vi "TEST Registry With Units.vi"() -> ()   [LabVIEW 2013, in "Carya Config.lvclass"]
doc: "Copyright 2018, Carya Automatisering, Wiebe Walstra."
uses:
  Carya Config.lvclass
  CConfig Variant Accessor/CConfig Variant Accessor.lvclass
  <vilib>/Utility/VariantDataType/VariantType.lvlib
panel:
  out "data 2":csg
  out "variant 2":variant
  out "variant":variant
  out "Formatted Strings 2":string[](array[string])
  out "x 2":dbl
  out "x":dbl
  out "J Bevel_cap height (m)":dbl[unit]
  out "J Bevel_cap height (m)":dbl=1.0
  in  "J Bevel_cap height (m)":dbl[unit]=0.001
  out "String 2":string
  out "Formatted Strings":string[](array[string])
  out "Numeric":cxt
  out "data":T1
  out "error out":errorcluster
  out "String":string
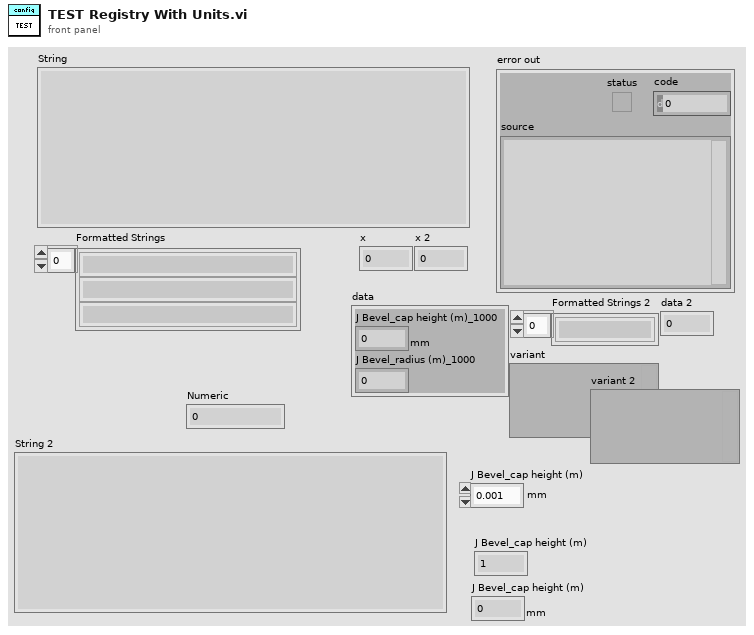
[diagram p1: front panel]
types:
  T1 = cluster{"J Bevel_cap height (m)_1000":dbl[unit], "J Bevel_radius (m)_1000":dbl}
  T2 = cluster{"J Bevel_cap height (m)_1000":dbl[unit], "J Bevel_cap height (m)_1000 2":dbl[unit], "J Bevel_cap height (m)_1000 3":dbl[unit]}
  T3 = cluster{"J Bevel_cap height (m)_1000":dbl, "J Bevel_radius (m)_1000":dbl}
  T4 = typedef "VariantType.lvlib/UnitInfo.ctl" = cluster{"UnitType":T5, "Exponent":i16}
  T5 = typedef "VariantType.lvlib/UnitType.ctl" = enum16{"Radians", "Steradians", "Seconds", "Meters", "Kilograms", "Amperes", "Kelvins", "Moles", "Candelas", "InvalidUnit"}
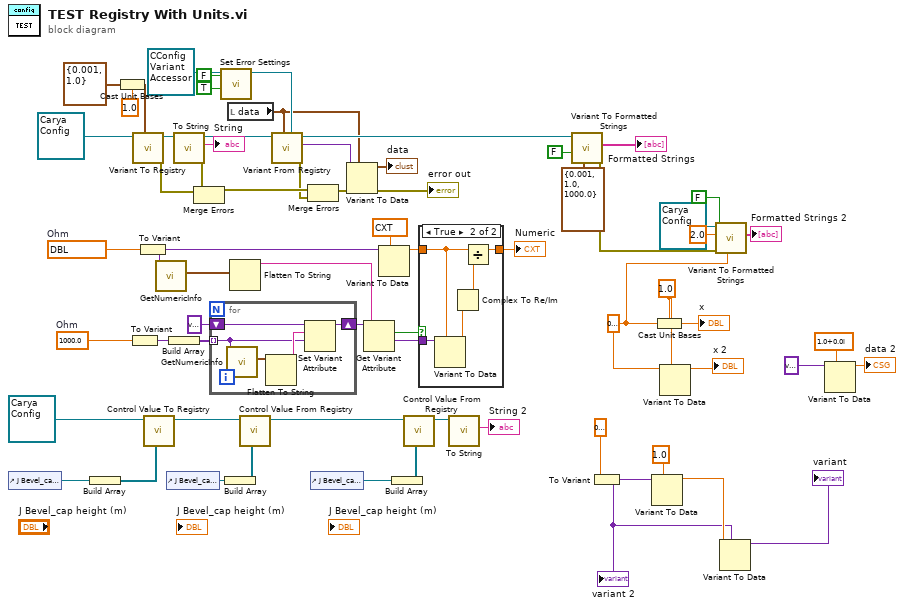
[diagram p0: block diagram]
diagram:
  w17 = 1.0 ("unit (none)")
  w15 = dbl[unit] 0.001 ("J Bevel_cap height (m)")
  w37 = dbl[unit] 1000.0  # Ohm
  w46 = cxt[unit] 100.0+200.0i  # Ohm
  n1 = control-ref of="J Bevel_cap height (m)"() -> (w29:refnum<vi>)
  n2 = Build Array(w29) -> (w28:refnum<vi>[])
  n3 = Cast Unit Bases(0:T1 {"J Bevel_cap height (m)_1000"=0.001, "J Bevel_radius (m)_1000"=1.0} ("J weld bevel"), 1:1.0) -> (2:w21:T3)
  n4 = To Variant(anything=w37) -> (Variant=w45:variant)
  n5 = call "Variant To Registry.vi"("Variant"=w21, "Carya Config in"=refnum<class "Carya Config.lvclass"> refnum) -> ("error out"=w62:errorcluster, "Carya Config out"=w66:refnum<class "Carya Config.lvclass">)  [unwired: 6 in, 2 out]
  n6 = To Variant(anything=w46) -> (Variant=w44:variant)
  n7 = call "Control Value To Registry.vi"("Controls"=w28, "Registry Object in"=refnum<class "Carya Config.lvclass"> refnum ("Carya Config in")) -> ("Registry Object out"=w30:refnum<class "Carya Config.lvclass">)  [unwired: 5 in, 4 out]
  n8 = call <vilib>:"GetNumericInfo.vi"("Variant"=w44) -> ("Units"=w41:T4[])  [unwired: 7 in, 3 out]
  n9 = control-ref of="J Bevel_cap height (m)"() -> (w27:refnum<vi>)
  n10 = Build Array(w45) -> (w47:variant[])
  n11 = call-dynamic "To String.vi"("Carya Config in"=w66) -> ("error out"=w63:errorcluster, "String"=→"String":string, "Carya Config out"=w64:refnum<class "Carya Config.lvclass">)  [unwired: 8 in]
  n12 = Merge Errors(w62, w63) -> (w61:errorcluster)
  n13 = for {
    tunnel: w47 -> [w69] mode=indexing
    shift-right: [w67] -> w42
    shift-left: variant -> [w68]
    n14 = call <vilib>:"GetNumericInfo.vi"("Variant"=w69) -> ("Units"=w71:T4[])  [unwired: 7 in, 3 out]
    n15 = Flatten To String(anything=w71) -> (data string=w70:string)  [unwired: 3 in, 2 out]
    n16 = Set Variant Attribute(Variant=w68, name=w70, value=w69) -> (Variant out=w67:variant)  [unwired: 1 in, 2 out]
  }
  n17 = call "Set Error Settings.vi"("Key not found error [F]"=TRUE ("Key not found error [T]"), "Wrong label error [F]"=FALSE, "CConfig Variant Accessor in"=refnum<class "CConfig Variant Accessor.lvclass"> refnum) -> ("CConfig Variant Accessor out"=w55:refnum<class "CConfig Variant Accessor.lvclass">)  [unwired: 7 in, 1 out]
  n18 = Build Array(w27) -> (w26:refnum<vi>[])
  n19 = local read "data"() -> (w20:T1)
  n20 = Flatten To String(anything=w41) -> (data string=w40:string)  [unwired: 3 in, 2 out]
  n21 = call "Control Value From Registry.vi"("Controls"=w26, "Registry Object in"=w30) -> ("Registry Object out"=w23:refnum<class "Carya Config.lvclass">)  [unwired: 7 in, 2 out]
  n22 = call "Variant From Registry.vi"("Registry Variant Accessor in"=w55, "Variant"=w20, "Carya Config in"=w64) -> ("error out"=w60:errorcluster, "Variant"=w59:variant, "Carya Config out"=w35:refnum<class "Carya Config.lvclass">)  [unwired: 5 in, 1 out]
  n23 = Merge Errors(w61, w60) -> (w58:errorcluster)
  n24 = control-ref of="J Bevel_cap height (m)"() -> (w24:refnum<vi>)
  n25 = Variant To Data(error in=w58, type=w20, Variant=w59) -> (data=→"data":T1, error out=→"error out":errorcluster)
  n26 = Get Variant Attribute(Variant=w42, name=w40) -> (found=w38:bool, value=w39:variant)  [unwired: 2 in, 2 out]
  n27 = Variant To Data(type=cxt 0.0+0.0i, Variant=w44) -> (data=w49:cxt)  [unwired: 1 in, 1 out]
  n28 = Build Array(w24) -> (w25:refnum<vi>[])
  n29 = call "Control Value From Registry.vi"("Controls"=w25, "Registry Object in"=w23) -> ("Registry Object out"=w22:refnum<class "Carya Config.lvclass">)  [unwired: 7 in, 2 out]
  n30 = case shown="True" w38 {
    tunnel: w49 -> [w72 w74]
    tunnel: [w72 w76] -> w48
    tunnel: w39 -> [_ w75]
    frame False {
    }
    frame True {
      n31 = Variant To Data(type=w74, Variant=w75) -> (data=w77:cxt)  [unwired: 1 in, 1 out]
      n32 = Complex To Re/Im(x + iy=w77) -> (x=w73:ext)  [unwired: 1 out]
      n33 = Divide(x=w74, y=w73) -> (x/y=w76:cxt)
    }
  }
  "Numeric" <- w48
  n34 = call-dynamic "To String.vi"("Carya Config in"=w22) -> ("String"=→"String 2":string)  [unwired: 8 in, 2 out]
  n35 = call "Variant To Formatted Strings.vi"("Variant"=T2 {"J Bevel_cap height (m)_1000"=0.001, "J Bevel_cap height (m)_1000 2"=1.0, "J Bevel_cap height (m)_1000 3"=1000.0}, "Read values? [T]"=FALSE, "Carya Config in"=w35) -> ("error out"=w4:errorcluster, "Formatted Strings"=→"Formatted Strings":string[])  [unwired: 5 in, 2 out]
  n36 = To Variant(anything=dbl[unit] 0.001 ("J Bevel_cap height (m)")) -> (Variant=w8:variant)
  "variant 2" <- w8
  n37 = Variant To Data(type=1.0 ("unit (none)"), Variant=w8) -> (data=w10:dbl)  [unwired: 1 in, 1 out]
  n38 = Cast Unit Bases(0:w15, 1:w17) -> (2:→"x":dbl)
  n39 = Variant To Data(type=w17, Variant=w15) -> (data=→"x 2":dbl)  [unwired: 1 in, 1 out]
  n40 = call "Variant To Formatted Strings.vi"("Variant"=w15, "error in (no error)"=w4, "Read values? [T]"=FALSE, "Multiply"=2.0 ("unit (none)"), "Carya Config in"=refnum<class "Carya Config.lvclass"> refnum) -> ("Formatted Strings"=→"Formatted Strings 2":string[])  [unwired: 3 in, 3 out]
  n41 = Variant To Data(type=w8, Variant=w10) -> (data=→"variant":variant)  [unwired: 1 in, 1 out]
  n42 = Variant To Data(type=csg 1.0+0.0i ("unit (none)"), Variant=variant ("variant")) -> (data=→"data 2":csg)  [unwired: 1 in, 1 out]
